vi "NI 5772 (AC) - DDC with IDL v1.8.vi"() -> ()   [LabVIEW 2015, in "DDC_7976R_v1.lvlib"]
doc: "Example Description:\nThis example demonstrates how to enable Time Interleaved Sampling with the NI 5772 adapter module to achieve a sampling rate of 1.6GS/s. This example continuously acquires records of analog input data from the NI 5772 adapter module. It allows you to select an AI channel, trigger type, and record size. This VI must be compiled before it is run. \n\nRunning the VI:\nThis VI must be run from the NI 5772 - Getting Started (Host).vi. Refer to the host VI documentation for steps regarding running and configuring the FPGA VI. \n\nExecution Steps:\nRefer to the Block Diagram of this VI for execution comments."
uses:
  DDC_7976R_v1.lvlib
  <instrlib>/_niInstr/DSP/v1/Shared/Public/IQ Gain.ctl
  <instrlib>/_niInstr/DSP/v1/Shared/Public/IQ Data.ctl
  <vilib>/Platform/TimedLoop/XDataNode/timing_clust.ctl
  <vilib>/Platform/TimedLoop/XDataNode/nitl_modes.ctl
  <vilib>/Platform/TimedLoop/XDataNode/wakeup.ctl
  <vilib>/rvi/Emulation/niFpgaGetClockAttributes.vi
  <vilib>/rvi/Emulation/niFpgaSctlEmulationGetInTimedLoop.vi
  <vilib>/rvi/Emulation/niFpgaEmulationReportErrorSimple.vi
  <vilib>/rvi/eio/common/nirviEmuTemplateMethod_errors.vi
  <vilib>/rvi/Emulation/niFpgaCriticalErrorInLSC.vi
  <instrlib>/_niInstr/DSP/v1/FPGA/Public/Sub VIs/Digital Gain/Digital Gain Base.vi
  <instrlib>/_niInstr/Basic Elements/v1/FPGA/Private/Count Up U64.vi
  <instrlib>/_niInstr/DSP/v1/FPGA/Public/Sub VIs/Frequency Shift/Frequency Shift - 8 spc.vi
  <vilib>/rvi/Emulation/niFpgaProcessEmulError.vi
  <instrlib>/_niInstr/DSP/v1/FPGA/Public/Sub VIs/HB Decimator/Halfband Decimator - IQ - 16 spc - 2x oc.vi
  <instrlib>/_niInstr/DSP/v1/FPGA/Public/Sub VIs/HB Decimator/Halfband Decimator - IQ - 8 spc - 2x oc.vi
  <instrlib>/_niInstr/DSP/v1/FPGA/Public/Sub VIs/HB Decimator/Halfband Decimator - IQ - 4 spc - 2x oc.vi
  <instrlib>/_niInstr/DSP/v1/FPGA/Public/Sub VIs/HB Decimator/Halfband Decimator - IQ - 2 spc - 2x oc.vi
  <instrlib>/_niInstr/DSP/v1/FPGA/Public/Sub VIs/Fractional Decimator/Fractional Decimator - 1 spc - 2x oc.vi
  <vilib>/eio/EIONode/EIONode.xnode
  <vilib>/Platform/TimedLoop/XDataNode/XDataNode.xnode
  <instrlib>/_niInstr/DSP/v1/Xnodes/Public/Digital Gain/niInstr DSP v1 Digital Gain FPGA.xnode
  <instrlib>/_niInstr/DSP/v1/Xnodes/Public/Frequency Shift/niInstr DSP v1 Frequency Shift FPGA.xnode
  <instrlib>/_niInstr/DSP/v1/Xnodes/Public/Decimator/niInstr DSP v1 Decimator FPGA.xnode
  <vilib>/Platform/TimedLoop/XDataNode/XDNodeRunTimeDep.lvlib
  <instrlib>/_niInstr/DSP/v1/Shared/niInstr DSP v1 Shared.lvlib
  <instrlib>/_niInstr/Basic Elements/v1/FPGA/niInstr Basic Elements v1 FPGA.lvlib
  <instrlib>/_niInstr/DSP/v1/FPGA/niInstr DSP v1 FPGA.lvlib
panel:
  in  "dbg.auth.pass":u64
  out "dbg.lic.error":bool
  in  "dbg.auth.code":u64
  in  "dbg.stream.enable.2":bool=TRUE
  in  "dbg.stream.enable.1":bool=TRUE
  out "dbg.cntr.rdy_f_in":u64
  out "dbg.cntr.2b":u64
  out "dbg.cntr.1b":u64
  out "dbg.2":T1
  out "dbg.cntr.5":u64
  out "dbg.cntr.4":u64
  out "dbg.cntr.3":u64
  out "dbg.cntr.2":u64
  out "dbg.cntr.1":u64
  out "dbg.1":T1[](array[typedef])
  in  "ddc.delay":fxp<+/-,16,0>[](array[numeric])=[0.0, 0.0, 0.0, 0.0, 0.0, 0.0, 0.0, 0.0, 0.0, 0.0, 0.0, 0.0, 0.0, 0.0, 0.0, 0.0]
  out "fifo.0.of":bool
  in  "ddc.out.rate":fxp<+,48,1>[](array[numeric])=[0.0, 0.0, 0.0, 0.0, 0.0, 0.0, 0.0, 0.0, 0.0, 0.0, 0.0, 0.0, 0.0, 0.0, 0.0, 0.0]
  in  "ddc.phase":fxp<+/-,21,0>[](array[numeric])=[0.0, 0.0, 0.0, 0.0, 0.0, 0.0, 0.0, 0.0, 0.0, 0.0, 0.0, 0.0, 0.0, 0.0, 0.0, 0.0] format="%#_21g"
  in  "ddc.freq.shift":fxp<+/-,48,0>[](array[numeric])=[0.0, 0.0, 0.0, 0.0, 0.0, 0.0, 0.0, 0.0, 0.0, 0.0, 0.0, 0.0, 0.0, 0.0, 0.0, 0.0]
  out "ddc.number.of.ch":u8
  out "ver.editorial":u8
  out "ver.technical":u8=1
  out "ver.major":u8=1
  in  "trig.samples.to.acq":u64
  in  "mode.continuous":bool
  out "dma.overflow":bool
  out "dsp.overflow":bool
  in  "input.gain":T2={"gain I"=1.0, "gain Q"=1.0}
  in  "trig.sw start trigger":bool
  in  "acq.reset":bool
  in  "User Command Commit":bool
  in  "User Command":u8
  out "User Command Idle":bool
  out "User Command Status":u8
  in  "User Data 0":u16
  in  "User Data 1":u8
  out "PLL Locked":bool
  out "User Error":bool
  out "Configured?":bool
  # "Refer to the Block Diagram of this VI for execution comments."
  # "Debug"
  # "For other instructions, select Help>>Show Context Help and move the cursor over the VI icon to display help for this VI."
  # "Resource Configuration"
  # "Trigger"
  # "Analog Input"
  # "Clock Configuration"
  # "DDC"
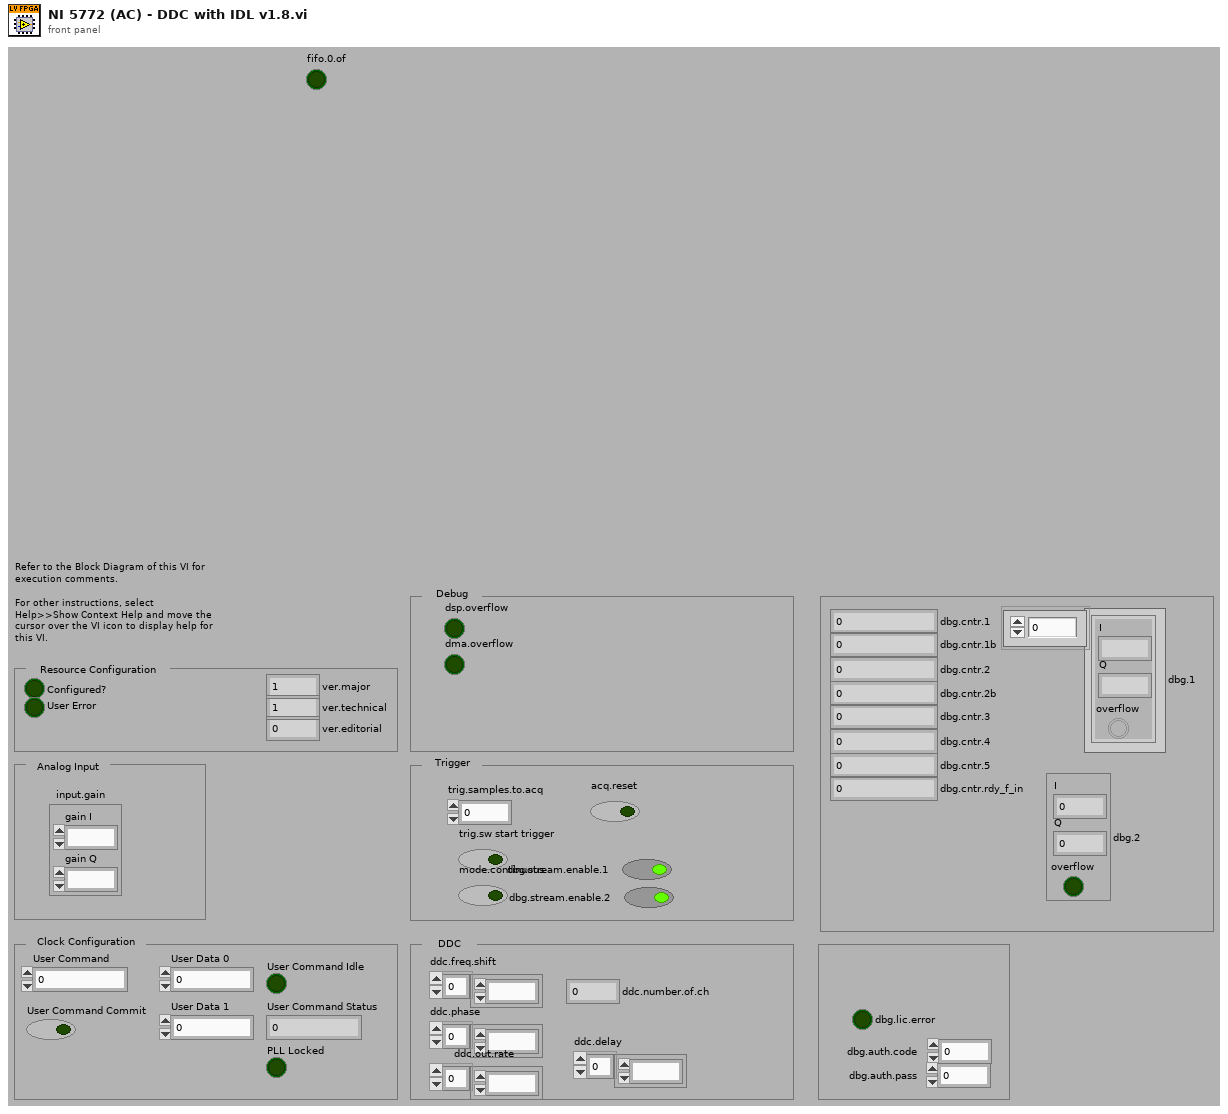
[diagram p1: front panel]
types:
  T1 = typedef "niInstr DSP v1 Shared.lvlib/IQ Data.ctl" = cluster{"I":fxp<+/-,18,1>, "Q":fxp<+/-,18,1>, "overflow":bool}
  T2 = typedef "niInstr DSP v1 Shared.lvlib/IQ Gain.ctl" = cluster{"gain I":fxp<+/-,24,3>, "gain Q":fxp<+/-,24,3>}
  T3 = typedef "XDNodeRunTimeDep.lvlib/timing_clust.ctl" = cluster{"Expected End [f-1]":u64, "Actual End [f-1]":u64, "Finished Late? [f-1]":bool, "Expected End [i-1]":u64, "Actual End [i-1]":u64, "Finished Late? [i-1]":bool, "Expected Start [i]":u64, "Actual Start [i]":u64, "Expected Start [f]":u64, "Actual Start [f]":u64, "Source Name":string, "Structure Name":string, "Period":i64, "Deadline":i64, "Offset":i64, "Start":i64, "Priority":i32, "Timeout":i32, "Mode":T4, "Wakeup Reason":T5, "Error":errorcluster, "Source Type":string, "Secondary Source Type":string, "Global End Time":u64, "Global Start Time":u64, "Frame Duration":u64, "Iteration Duration":u64, "Assigned CPU":i32, "I/O Scan Engine Mode":u32}
  T4 = typedef "XDNodeRunTimeDep.lvlib/nitl_modes.ctl" = enum32{"No Change", "Process missed periods, maintain original phase", "Discard missed periods, maintain original phase", "Process missed periods, ignore original phase", "Discard missed periods, ignore original phase"}
  T5 = typedef "XDNodeRunTimeDep.lvlib/wakeup.ctl" = enum32{"Normal", "Aborted", "Asynchronous wakeup", "Timing source error", "Timed loop error", "Timeout"}
  T6 = cluster{"I":fxp<+/-,18,1>, "Q":fxp<+/-,18,1>, "overflow":bool}[]
  T7 = typedef "DDC_7976R_v1.lvlib/16xIQData.ctl" = T1[]
  T8 = typedef "DDC_7976R_v1.lvlib/16xIQData_without_overflow.ctl" = cluster{"I":fxp<+/-,18,1>, "Q":fxp<+/-,18,1>}[]
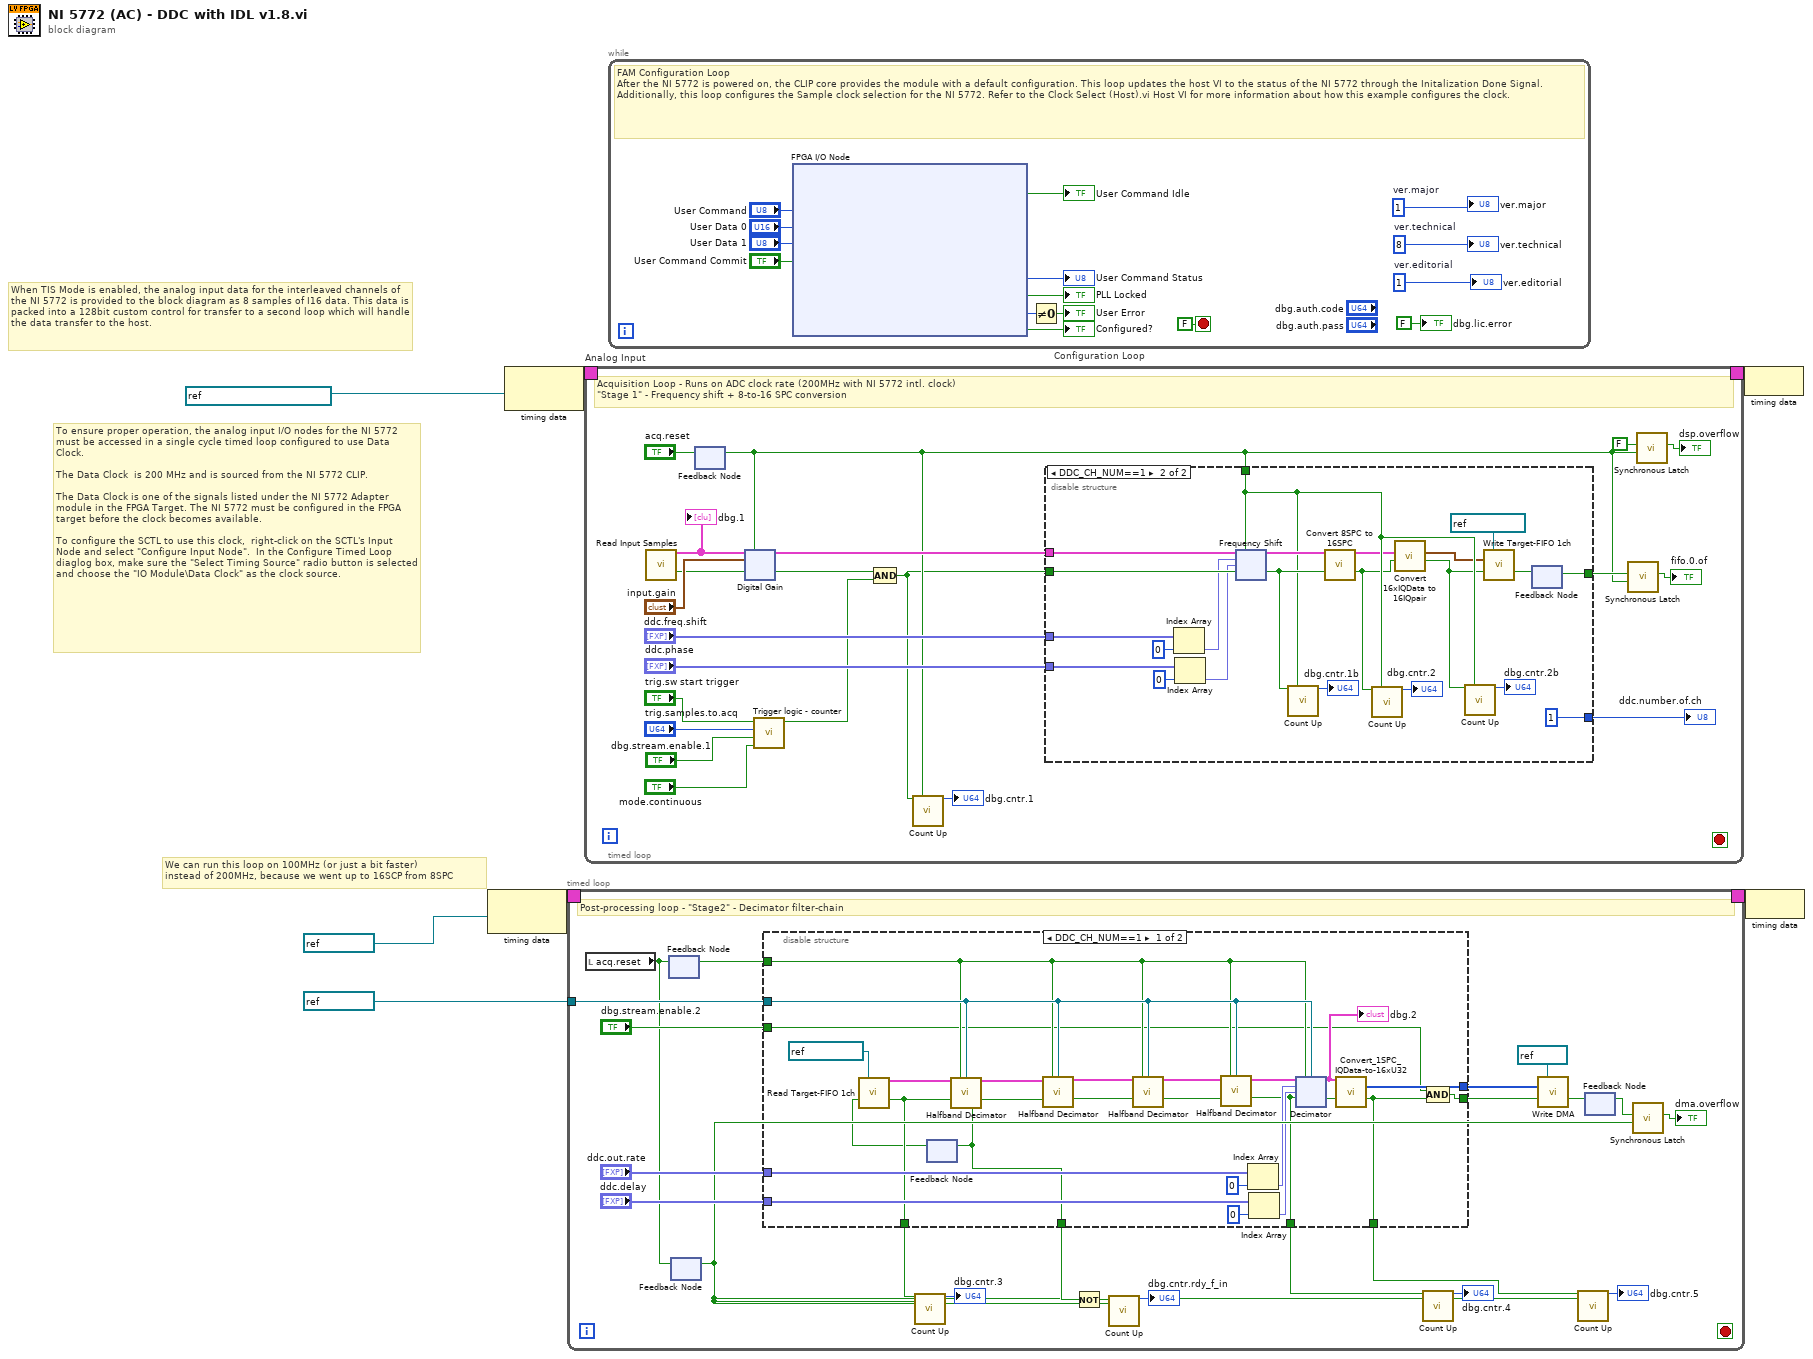
[diagram p0: block diagram]
diagram:
  # "We can run this loop on 100MHz (or just a bit faster)\ninstead of 200MHz, because we went up to 16SCP from 8SPC"
  # "When TIS Mode is enabled, the analog input data for the interleaved channels of the NI 5772 is provided to the block diagram as 8 samples of I16 data. This data is packed into a 128bit custom control for transfer to a second loop which will handle the data transfer to the host."
  # "To ensure proper operation, the analog input I/O nodes for the NI 5772 must be accessed in a single cycle timed loop configured to use Data Clock. \n\nThe Data Clock  is 200 MHz and is sourced from the NI 5772 CLIP.\n\nThe Data Clock is one of the signals listed under the NI 5772 Adapter module in the FPGA Target. The NI 5772 must be configured in the FPGA target before the clock becomes available. \n\nTo configure the SCTL to use this clock,  right-click on the SCTL's Input Node and select \"Configure Input Node\".  In the Configure Timed Loop diaglog box, make sure the \"Select Timing Source\" radio button is selected and choose the \"IO Module\\Data Clock\" as the clock source."
  n1 = node-c288(refnum<k21> "102MHz" ("Source Name")) -> (w4:T3)
  n2 = node-c288(refnum<k21> "IO Module\\Data Clock" ("Source Name")) -> (w7:T3)
  n3 = timed-loop {
    timing: w4 -> [_]
    timing-out: [_] -> w3
    tunnel: refnum<k21> "204MHz" ("Source Name") -> [w27]
    stop <- _ stop-if-true
    # "Post-processing loop - \"Stage2\" - Decimator filter-chain"
    n4 = local read "acq.reset"() -> (w13:bool)
    n5 = feedback #1() -> (w16:bool)  [unwired: 1 in]
    n6 = feedback-in #1(w13) -> ()
    n7 = feedback #2() -> (w12:bool)  [unwired: 1 in]
    n8 = feedback-in #2(w13) -> ()
    n9 = disable-structure shown="DDC_CH_NUM==1" {
      disable-tunnel: w27 -> [w49 _]
      disable-tunnel: "ddc.out.rate" -> [w48 _]
      disable-tunnel: "ddc.delay" -> [w45 _]
      disable-tunnel: [w42 _] -> w23
      disable-tunnel: [w41 _] -> w21
      disable-tunnel: [w39 _] -> w18
      disable-tunnel: w16 -> [w38 _]
      disable-tunnel: "dbg.stream.enable.2" -> [w30 _]
      disable-tunnel: [w33 _] -> w14
      disable-tunnel: [w32 _] -> w10
      disable-tunnel: [w31 _] -> w9
      frame condition #0 (active) {
        n10 = feedback #3() -> (w37:bool)  [unwired: 1 in]
        n11 = call "Read Target-FIFO 1ch.vi"("FIFO In"=refnum<k21> "FIFO-000", "ready for input"=w37) -> ("16xIQData"=w40:T6, "Output Valid"=w42:bool)  [unwired: 12 in]
        n12 = call-poly <instrlib>:"Halfband Decimator.vi"("data in"=w40, "reset"=w38, "clock x 2"=w49, "input valid"=w42) -> ("data out"=w56:T1[], "output valid"=w55:bool, "ready for input"=w39:bool)  [unwired: 9 in]
        n13 = feedback-in #3(w39) -> ()
        n14 = call-poly <instrlib>:"Halfband Decimator.vi"("data in"=w56, "reset"=w38, "clock x 2"=w49, "input valid"=w55) -> ("data out"=w54:T1[], "output valid"=w53:bool)  [unwired: 9 in, 1 out]
        n15 = call-poly <instrlib>:"Halfband Decimator.vi"("data in"=w54, "reset"=w38, "clock x 2"=w49, "input valid"=w53) -> ("data out"=w52:T1[], "output valid"=w50:bool)  [unwired: 9 in, 1 out]
        n16 = call-poly <instrlib>:"Halfband Decimator.vi"("data in"=w52, "reset"=w38, "clock x 2"=w49, "input valid"=w50) -> ("data out"=w51:T1, "output valid"=w41:bool)  [unwired: 9 in, 1 out]
        n17 = Index Array(array=w48, index=0) -> (element=w43:fxp<+,48,1>)
        n18 = Index Array(array=w45, index=0) -> (element=w44:fxp<+/-,16,0>)
        n19 = xnode "Decimator"("data in"=w51, "reset"=w38, "input valid"=w41, "output sample rate"=w43, "delay"=w44, "clock x2"=w49) -> ("data out"=w35:T1, "output valid"=w34:bool)  [unwired: 1 out]
        "dbg.2" <- w35
        n20 = call "Convert_1SPC_IQData-to-16xU32.vi"("1SPC-IQ in"=w35, "Input valid"=w34) -> ("16xU32"=w32:u32[], "Output valid"=w33:bool)  [unwired: 11 in, 1 out]
        n21 = Compound Arithmetic op=AND(w30, w33) -> (w31:bool)
      }
      frame condition #1 {
      }
    }
    n22 = call-poly <instrlib>:"Count Up.vi"("increment"=w23, "reset"=w12) -> ("count out"=→"dbg.cntr.3":u64)  [unwired: 13 in]
    n23 = Not(x=w18) -> (.not. x?=w17:bool)
    n24 = call-poly <instrlib>:"Count Up.vi"("increment"=w17, "reset"=w12) -> ("count out"=→"dbg.cntr.rdy_f_in":u64)  [unwired: 13 in]
    n25 = call-poly <instrlib>:"Count Up.vi"("increment"=w21, "reset"=w12) -> ("count out"=→"dbg.cntr.4":u64)  [unwired: 13 in]
    n26 = call "Write DMA.vi"("FIFO In"=refnum<k21> "T2H", "16xU32"=w10, "input valid"=w9) -> ("Timed Out?"=w8:bool)  [unwired: 12 in]
    n27 = call-poly <instrlib>:"Count Up.vi"("increment"=w14, "reset"=w12) -> ("count out"=→"dbg.cntr.5":u64)  [unwired: 13 in]
    n28 = feedback #4() -> (w29:bool)  [unwired: 1 in]
    n29 = feedback-in #4(w8) -> ()
    n30 = call <instrlib>:"Synchronous Latch.vi"("clear"=w12, "set"=w29) -> ("out"=→"dma.overflow":bool)  [unwired: 9 in]
  }
  n31 = timed-loop "Analog Input" {
    timing: w7 -> [_]
    timing-out: [_] -> w6
    stop <- _ stop-if-true
    # "Acquisition Loop - Runs on ADC clock rate (200MHz with NI 5772 intl. clock)\n\"Stage 1\" - Frequency shift + 8-to-16 SPC conversion"
    n32 = call "Read Input Samples.vi"() -> ("Array"=w83:T1[], "output valid"=w75:bool)  [unwired: 14 in]
    "dbg.1" <- w83
    n33 = feedback #5() -> (w72:bool)  [unwired: 1 in]
    n34 = feedback-in #5("acq.reset") -> ()
    n35 = xnode "Digital Gain"("data in"=w83, "reset"=w72, "gain"="input.gain", "input valid"=w75) -> ("data out"=w81:T1[], "output valid"=w70:bool)  [unwired: 1 in, 1 out]
    n36 = call "Trigger logic - counter.vi"("mode.continuous"="mode.continuous", "stream.enable"="dbg.stream.enable.1", "trig.samples.to.acq"="trig.samples.to.acq", "trig.sw start trigger"="trig.sw start trigger") -> ("enable out"=w71:bool)  [unwired: 7 in]
    n37 = Compound Arithmetic op=AND(w70, w71) -> (w69:bool)
    n38 = call-poly <instrlib>:"Count Up.vi"("increment"=w69, "reset"=w72) -> ("count out"=→"dbg.cntr.1":u64)  [unwired: 13 in]
    n39 = disable-structure shown="DDC_CH_NUM==1" {
      disable-tunnel: [_ u8 1] -> w82
      disable-tunnel: w81 -> [_ w109]
      disable-tunnel: w69 -> [_ w108]
      disable-tunnel: w72 -> [_ w93]
      disable-tunnel: "ddc.freq.shift" -> [_ w106]
      disable-tunnel: "ddc.phase" -> [_ w105]
      disable-tunnel: [_ w99] -> w76
      frame condition #0 {
      }
      frame condition #1 (active) {
        n40 = Index Array(array=w106, index=0) -> (element=w102:fxp<+/-,48,0>)
        n41 = Index Array(array=w105, index=0) -> (element=w101:fxp<+/-,21,0>)
        n42 = xnode "Frequency Shift"("data in"=w109, "reset"=w93, "frequency shift"=w102, "phase"=w101, "input valid"=w108) -> ("data out"=w107:T1[], "output valid"=w96:bool)  [unwired: 1 in, 1 out]
        n43 = call-poly <instrlib>:"Count Up.vi"("increment"=w96, "reset"=w93) -> ("count out"=→"dbg.cntr.1b":u64)  [unwired: 13 in]
        n44 = call "Convert 8SPC to 16SPC.vi"("8xIQ in"=w107, "input valid"=w96) -> ("16xIQ out"=w92:T7, "output valid"=w90:bool)  [unwired: 12 in]
        n45 = call-poly <instrlib>:"Count Up.vi"("increment"=w90, "reset"=w93) -> ("count out"=→"dbg.cntr.2":u64)  [unwired: 13 in]
        n46 = call "Convert 16xIQData to 16IQpair.vi"("input valid"=w90, "16xIQdata in"=w92) -> ("output valid"=w89:bool, "16xIQpair out"=w91:T8)  [unwired: 7 in, 1 out]
        n47 = call-poly <instrlib>:"Count Up.vi"("increment"=w89, "reset"=w93) -> ("count out"=→"dbg.cntr.2b":u64)  [unwired: 13 in]
        n48 = call "Write Target-FIFO 1ch.vi"("FIFO In"=refnum<k21> "FIFO-000", "16IQ in"=w91, "input valid"=w89) -> ("Timed Out?"=w100:bool)  [unwired: 12 in]
        n49 = feedback #6() -> (w99:bool)  [unwired: 1 in]
        n50 = feedback-in #6(w100) -> ()
      }
    }
    "ddc.number.of.ch" <- w82
    n51 = call <instrlib>:"Synchronous Latch.vi"("clear"=w72, "set"=w76) -> ("out"=→"fifo.0.of":bool)  [unwired: 9 in]
    n52 = call <instrlib>:"Synchronous Latch.vi"("clear"=w72, "set"=FALSE) -> ("out"=→"dsp.overflow":bool)  [unwired: 9 in]
  }
  n53 = while "Configuration Loop" {
    stop <- FALSE stop-if-true
    w162 = u8 1  # ver.editorial
    w163 = u8 8  # ver.technical
    w164 = u8 1  # ver.major
    # "FAM Configuration Loop\nAfter the NI 5772 is powered on, the CLIP core provides the module with a default configuration. This loop updates the host VI to the status of the NI 5772 through the Initalization Done Signal. Additionally, this loop configures the Sample clock selection for the NI 5772. Refer to the Clock Select (Host).vi Host VI for more information about how this example configures the clock."
    n54 = xnode "FPGA I/O Node"("IO Module\\User Command"="User Command", "IO Module\\User Data 0"="User Data 0", "IO Module\\User Data 1"="User Data 1", "IO Module\\User Command Commit"="User Command Commit") -> ("IO Module\\User Command Idle"=→"User Command Idle":bool, "IO Module\\User Command Status"=→"User Command Status":u8, "IO Module\\PLL Locked"=→"PLL Locked":bool, "IO Module\\User Error"=w170:u8, "IO Module\\Initialization Done"=→"Configured?":bool)  [unwired: 9 in, 9 out]
    n55 = Not Equal To 0?(x=w170) -> (x != 0?=→"User Error":bool)
    "ver.major" <- w164
    "ver.technical" <- w163
    "ver.editorial" <- w162
    "dbg.lic.error" <- FALSE ("dbg.lic.error")
  }
  n56 = node-c288(w6) -> ()
  n57 = node-c288(w3) -> ()
